vi "Save Values_UI.vi"(8 "error in (no error)":errorcluster, 10 "Controls and Indicators\nReferences":T1, 11 "Input ListBox Cluster":T7) -> (0 "error out":errorcluster, 3 "ListBox Cluster out":T7)   [LabVIEW 2019, in "ZenGage v3.0 UI.lvclass"]
doc: "This VI replaces entered Lower Limit, Upper Limit, Lower Control Limit, and Upper Control Limit in Measurement Listbox and Edit Measurement Listbox and then sends message to Save pressed_SM.vi."
uses:
  ZenGage v3.0 UI.lvclass
  Type Definitions/Edit tolerance settings/Rack Selection.ctl
  Type Definitions/Edit tolerance settings/Edit Tolerance Input.ctl
  <vilib>/Utility/miscctls.llb/LVPoint32TypeDef.ctl
  Type Definitions/Controls and Indicators/Select a part (combobox).ctl
  Type Definitions/Controls and Indicators/EDL control references.ctl
  Type Definitions/Controls and Indicators/Diagnostics control referencs.ctl
  Type Definitions/Controls and Indicators/Inspection control references.ctl
  Type Definitions/Controls and Indicators/General_Control references.ctl
  Type Definitions/Controls and Indicators/Controls and Indicators Cluster.ctl
  Type Definitions/General/Master sample references.ctl
panel:
  in  "Rack Number":i32
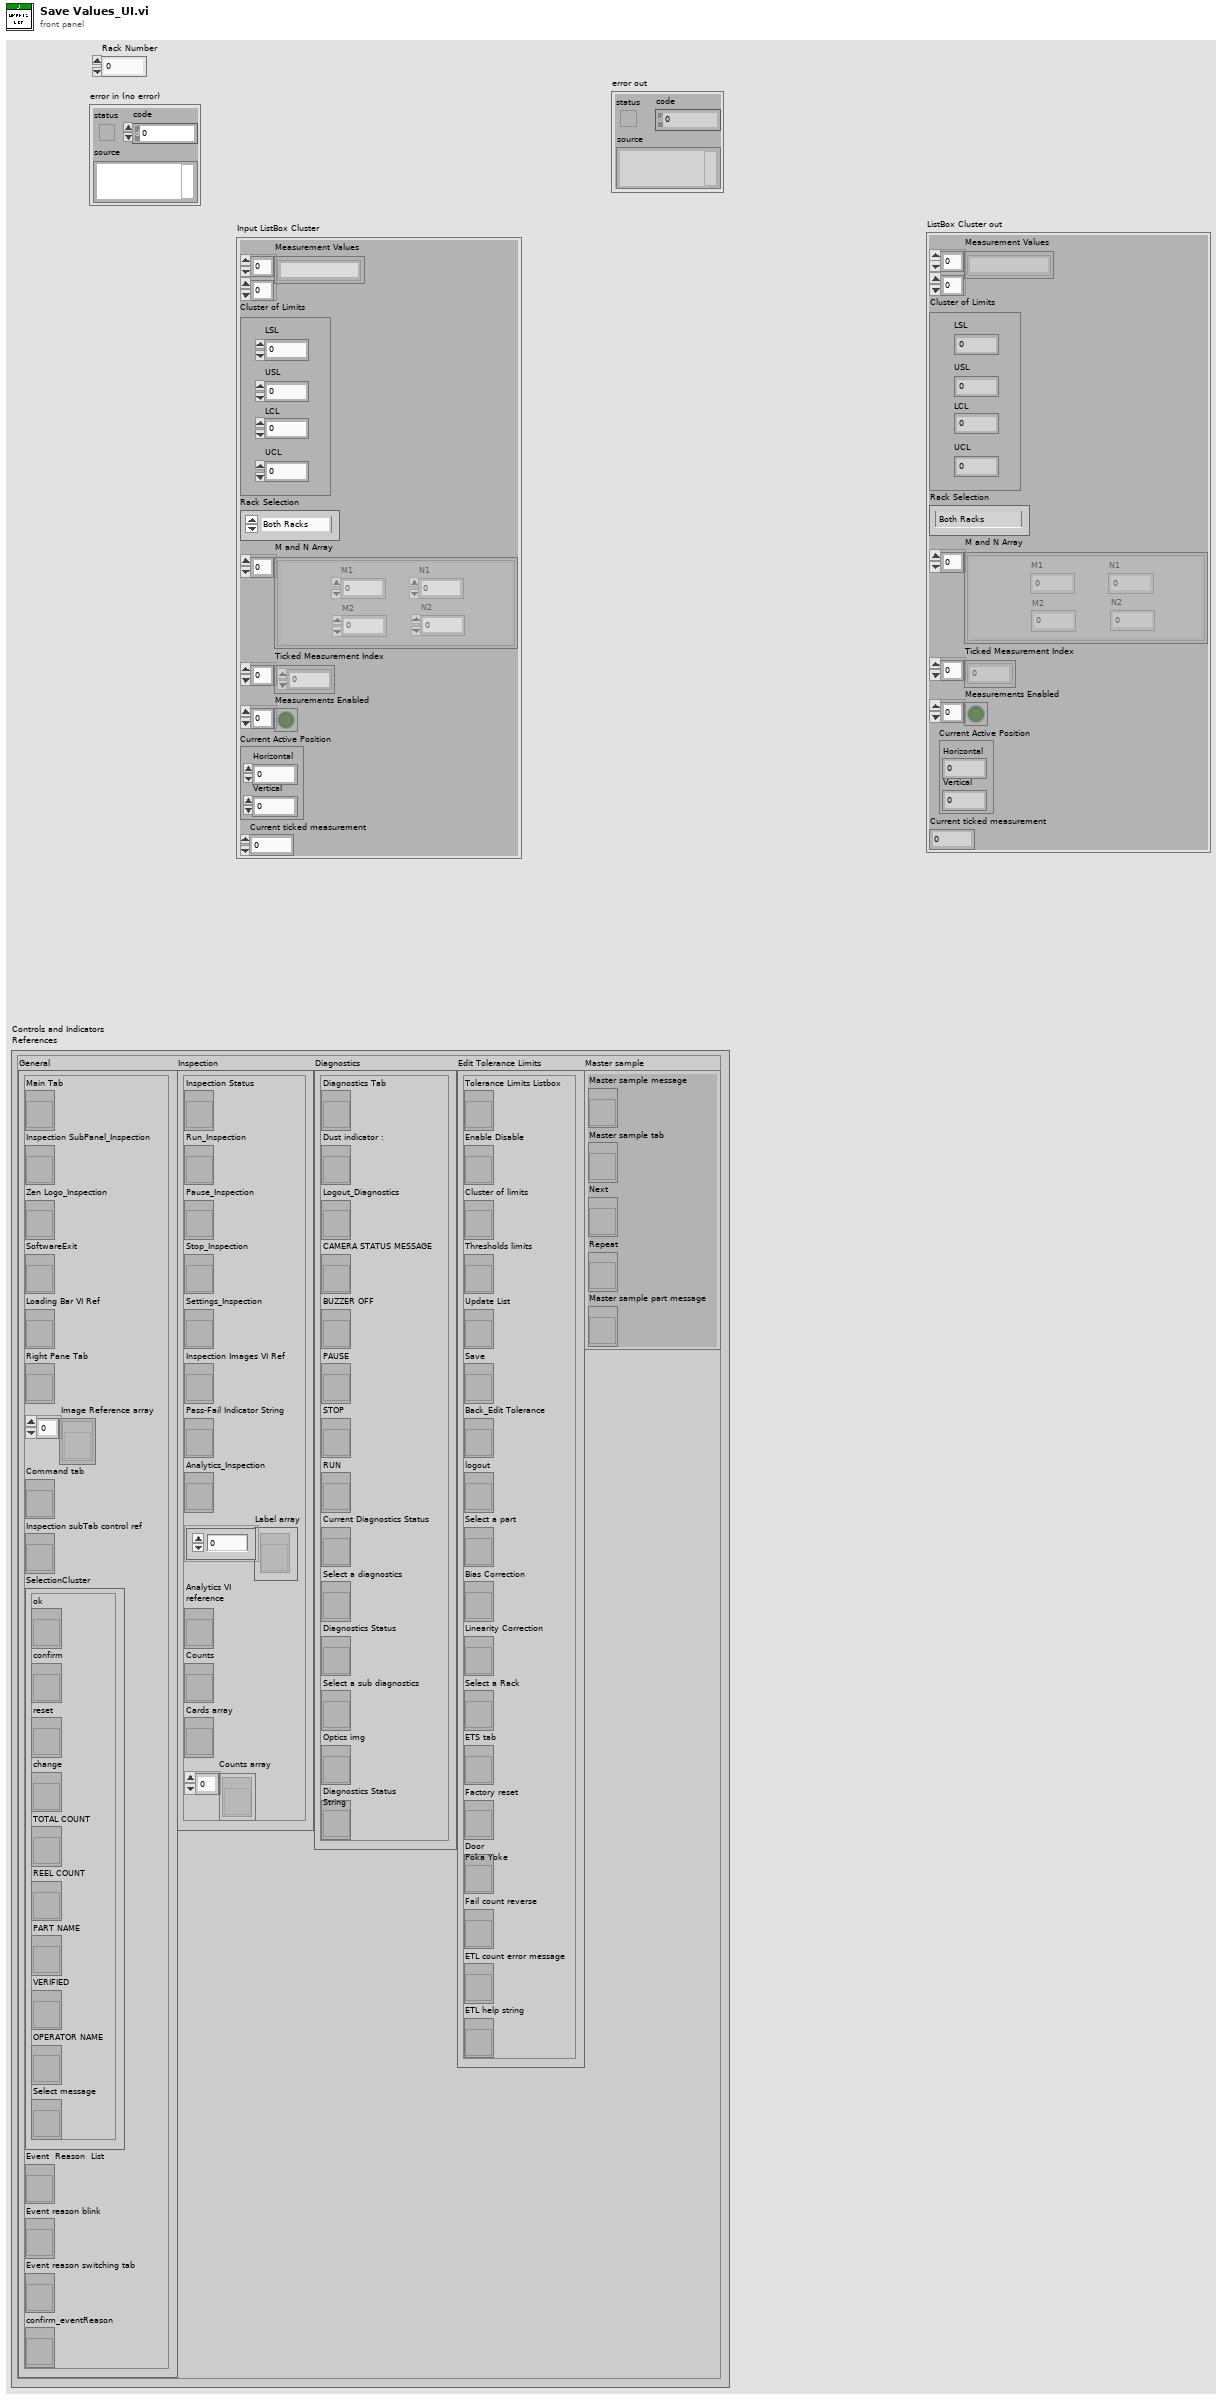
[diagram p1: front panel]
types:
  T1 = typedef "ZenGage v3.0 UI.lvclass/Controls and Indicators Cluster.ctl" = cluster{"General":T2, "Inspection":T3, "Diagnostics":T4, "Edit Tolerance Limits":T5, "Master sample":T6}
  T2 = typedef "ZenGage v3.0 UI.lvclass/General_Control references.ctl" = cluster{"Main Tab":refnum<vi>, "Inspection SubPanel_Inspection":refnum<vi>, "Zen Logo_Inspection":refnum<vi>, "SoftwareExit":refnum<vi>, "Loading Bar VI Ref":refnum<vi>, "Right Pane Tab":refnum<vi>, "Image Reference array":refnum<vi>[], "Command tab":refnum<vi>, "Inspection subTab control ref":refnum<vi>, "SelectionCluster":cluster{"ok":refnum<vi>, "confirm":refnum<vi>, "reset":refnum<vi>, "change":refnum<vi>, "TOTAL COUNT":refnum<vi>, "REEL COUNT":refnum<vi>, "PART NAME":refnum<vi>, "VERIFIED":refnum<vi>, "OPERATOR NAME":refnum<vi>, "Select message":refnum<vi>}, "Event  Reason  List":refnum<vi>, "Event reason blink":refnum<vi>, "Event reason switching tab":refnum<vi>, "confirm_eventReason":refnum<vi>}
  T3 = typedef "ZenGage v3.0 UI.lvclass/Inspection control references.ctl" = cluster{"Inspection Status":refnum<vi>, "Run_Inspection":refnum<vi>, "Pause_Inspection":refnum<vi>, "Stop_Inspection":refnum<vi>, "Settings_Inspection":refnum<vi>, "Inspection Images VI Ref":refnum<vi>, "Pass-Fail Indicator String":refnum<vi>, "Analytics_Inspection":refnum<vi>, "Label array":refnum<vi>[], "Analytics VI\nreference":refnum<vi>, "Counts":refnum<vi>, "Cards array":refnum<vi>, "Counts array":refnum<vi>[]}
  T4 = typedef "ZenGage v3.0 UI.lvclass/Diagnostics control referencs.ctl" = cluster{"Diagnostics Tab":refnum<vi>, "Dust indicator :":refnum<vi>, "Logout_Diagnostics":refnum<vi>, "CAMERA STATUS MESSAGE":refnum<vi>, "BUZZER OFF":refnum<vi>, "PAUSE":refnum<vi>, "STOP":refnum<vi>, "RUN":refnum<vi>, "Current Diagnostics Status":refnum<vi>, "Select a diagnostics":refnum<vi>, "Diagnostics Status":refnum<vi>, "Select a sub diagnostics":refnum<vi>, "Optics img":refnum<vi>, "Diagnostics Status\nString":refnum<vi>}
  T5 = typedef "ZenGage v3.0 UI.lvclass/EDL control references.ctl" = cluster{"Tolerance Limits Listbox":refnum<vi>, "Enable Disable":refnum<vi>, "Cluster of limits":refnum<vi>, "Thresholds limits":refnum<vi>, "Update List":refnum<vi>, "Save":refnum<vi>, "Back_Edit Tolerance":refnum<vi>, "logout":refnum<vi>, "Select a part":refnum<vi>, "Bias Correction":refnum<vi>, "Linearity Correction":refnum<vi>, "Select a Rack":refnum<vi>, "ETS tab":refnum<vi>, "Factory reset":refnum<vi>, "Door\nPoka Yoke":refnum<vi>, "Fail count reverse":refnum<vi>, "ETL count error message":refnum<vi>, "ETL help string":refnum<vi>}
  T6 = typedef "Master sample references.ctl" = cluster{"Master sample message":refnum<vi>, "Master sample tab":refnum<vi>, "Next":refnum<vi>, "Repeat":refnum<vi>, "Master sample part message":refnum<vi>}
  T7 = typedef "ZenGage v3.0 UI.lvclass/Edit Tolerance Input.ctl" = cluster{"Measurement Values":string[][], "Cluster of Limits":cluster{"LSL":dbl, "USL":dbl, "LCL":dbl, "UCL":dbl}, "Rack Selection":T8, "M and N Array":cluster{"M1":u64, "M2":u64, "N1":u64, "N2":u64}[], "Ticked Measurement Index":u32[], "Measurements Enabled":bool[], "Current Active Position":T9, "Current ticked measurement":dbl}
  T8 = typedef "ZenGage v3.0 UI.lvclass/Rack Selection.ctl" = enum16{"Both Racks", "Rack 2", "Rack 1"}
  T9 = typedef "LVPoint32TypeDef.ctl" = cluster{"Horizontal":i32, "Vertical":i32}
  T10 = enum8{"Enabled", "Disabled", "Disabled and Grayed Out"}
  T11 = cluster{"Lower Limit":dbl, "Upper Limit":dbl, "Lower Control Limit":dbl, "Upper Control Limit":dbl}
  T12 = cluster{"Control Limit Fail Allowable":u64, "Control Limit Fail Window":u64, "Spec Limit Fail Allowable":u64, "Spec Limit Fail Window":u64}
  T13 = cluster{"LSL":dbl, "USL":dbl, "LCL":dbl, "UCL":dbl}
  T14 = cluster{"M1":u64, "M2":u64, "N1":u64, "N2":u64}[]
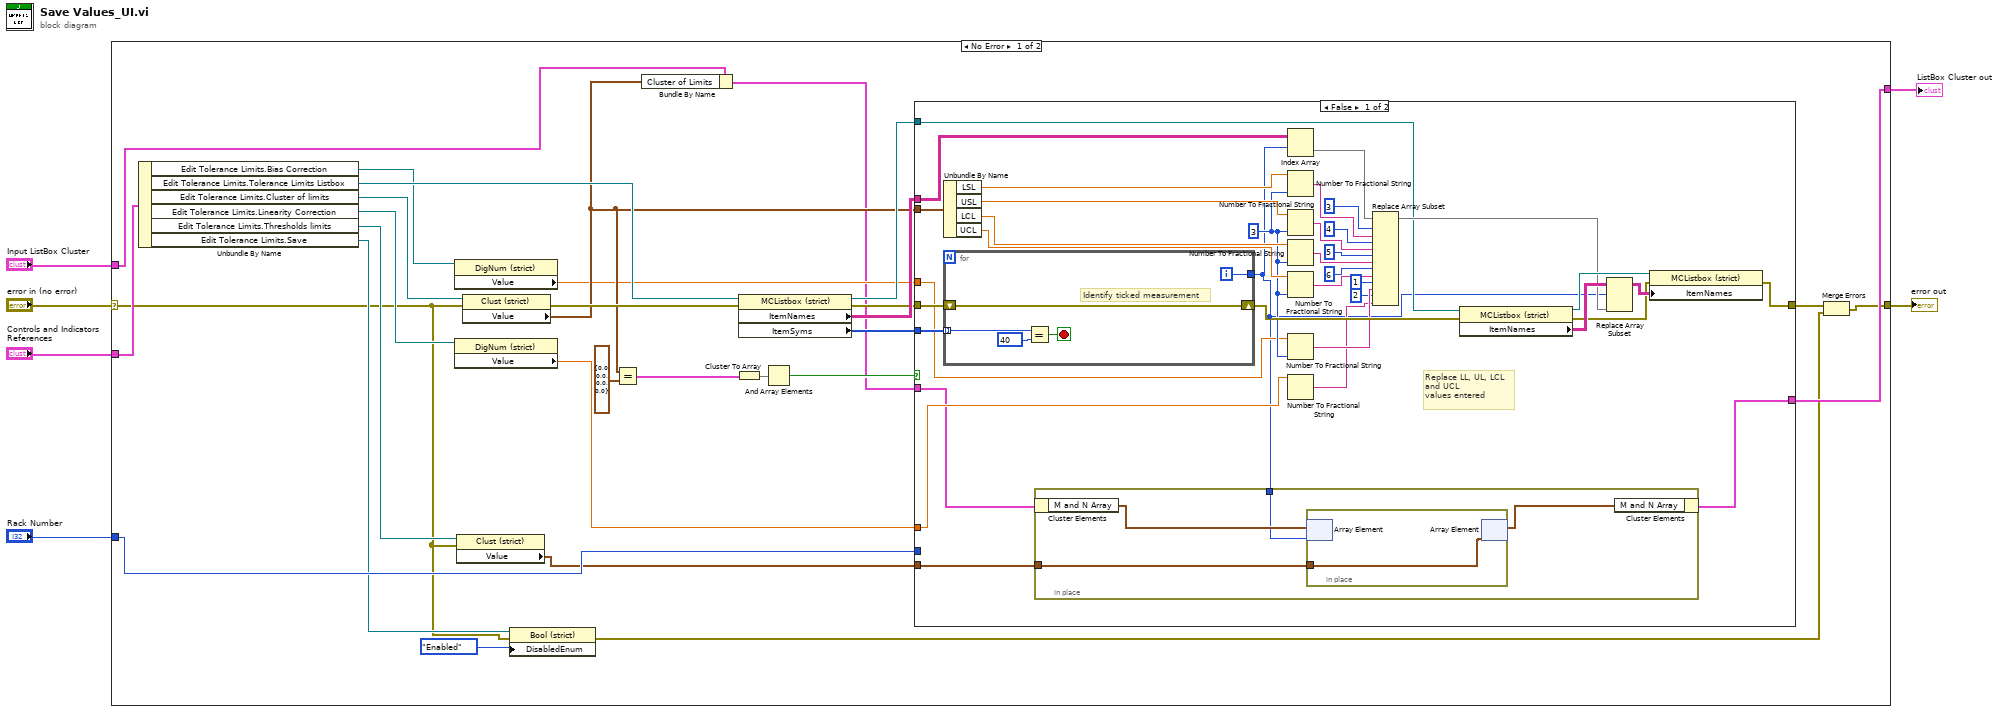
[diagram p0: block diagram]
diagram:
  n1 = case shown="No Error" "error in (no error)" {
    selector: "error in (no error)" -> [w10 w85]
    tunnel: [w7 w85] -> w5
    tunnel: "Input ListBox Cluster" -> [w13 w84]
    tunnel: [w14 w84] -> w3
    tunnel: "Rack Number" -> [w17 _]
    tunnel: "Controls and Indicators\nReferences" -> [w18 _]
    frame No Error {
      n2 = Unbundle By Name(w18) -> ("Edit Tolerance Limits.Bias Correction"=w23:refnum<vi>, "Edit Tolerance Limits.Tolerance Limits Listbox"=w25:refnum<vi>, "Edit Tolerance Limits.Cluster of limits"=w27:refnum<vi>, "Edit Tolerance Limits.Linearity Correction"=w21:refnum<vi>, "Edit Tolerance Limits.Thresholds limits"=w19:refnum<vi>, "Edit Tolerance Limits.Save"=w12:refnum<vi>)
      n3 = property class="DigNum (strict)"(reference=w23) -> ("Value"=w22:dbl)  [unwired: 1 in, 2 out]
      n4 = property class="DigNum (strict)"(reference=w21) -> ("Value"=w20:dbl)  [unwired: 1 in, 2 out]
      n5 = property class="Clust (strict)"(reference=w19, error in=w10) -> ("Value"=w16:T12)  [unwired: 2 out]
      n6 = property class="Clust (strict)"(reference=w27, error in=w10) -> (error out=w26:errorcluster, "Value"=w24:T13)  [unwired: 1 out]
      n7 = property class="Bool (strict)"(reference=w12, error in=w10, "DisabledEnum"=T10."Enabled" ("Disabled")) -> (error out=w8:errorcluster)  [unwired: 1 out]
      n8 = Equal?(x=w24, y=T11 {"Lower Limit"=0.0, "Upper Limit"=0.0, "Lower Control Limit"=0.0, "Upper Control Limit"=0.0} ("Value")) -> (x = y?=w33:cluster{bool, bool, bool, bool})
      n9 = Bundle By Name(cluster=w13, "Cluster of Limits"=w24) -> (w15:T7)
      n10 = Cluster To Array(cluster=w33) -> (array=w34:bool[])
      n11 = property class="MCListbox (strict)"(reference=w25, error in=w26) -> (reference out=w28:refnum<vi>, error out=w30:errorcluster, "ItemNames"=w31:string[][], "ItemSyms"=w29:i32[])
      n12 = And Array Elements(Boolean array=w34) -> (logical AND=w35:bool)
      n13 = case shown="False" w35 {
        tunnel: w29 -> [w71 _]
        tunnel: w28 -> [w40 _]
        tunnel: w30 -> [w51 w83]
        tunnel: [w49 w83] -> w9
        tunnel: w31 -> [w56 _]
        tunnel: w24 -> [w52 _]
        tunnel: w22 -> [w46 _]
        tunnel: w20 -> [w42 _]
        tunnel: w17 -> [_ _]
        tunnel: w16 -> [w39 _]
        tunnel: w15 -> [w37 w82]
        tunnel: [w36 w82] -> w14
        frame False {
          w47 = i16 3 ("precision (6)")
          # "Replace LL, UL, LCL \nand UCL\nvalues entered"
          n14 = Unbundle By Name(w52) -> ("LSL"=w69:dbl, "USL"=w68:dbl, "LCL"=w67:dbl, "UCL"=w66:dbl)
          n15 = for {
            tunnel: w71 -> [w80] mode=indexing
            tunnel: [w78] -> w38
            shift-right: [w77] -> w50
            shift-left: w51 -> [w77]
            i -> [w78]
            stop <- w79 stop-if-true
            # "Identify ticked measurement"
            n16 = Equal?(x=w80, y=40) -> (x = y?=w79:bool)
          }
          n17 = in-place {
            in-place-border: w39 -> [w75]
            in-place-border: w38 -> [w72]
            n18 = in-place-cluster #1(w37) -> ("M and N Array"=w74:T14)
            n19 = in-place {
              in-place-border: w75 -> [w76]
              n20 = in-place-array #2(w74, w72) -> ()  [unwired: 1 out]
              n21 = in-place-array #2(w76) -> (w73:T14)  [unwired: 1 out]
            }
            n22 = in-place-cluster #1("M and N Array"=w73) -> (w36:T7)
          }
          n23 = Index Array(array=w56, index (row)=w38) -> (element=w70:string[])  [unwired: 1 in]
          n24 = Number To Fractional String(number=w69, precision (6)=w47) -> (F-format string=w65:string)  [unwired: 2 in]
          n25 = Number To Fractional String(number=w68, precision (6)=w47) -> (F-format string=w64:string)  [unwired: 2 in]
          n26 = Number To Fractional String(number=w67, precision (6)=w47) -> (F-format string=w63:string)  [unwired: 2 in]
          n27 = Number To Fractional String(number=w66, precision (6)=w47) -> (F-format string=w62:string)  [unwired: 2 in]
          n28 = Number To Fractional String(number=w46, precision (6)=w47) -> (F-format string=w44:string)  [unwired: 2 in]
          n29 = Number To Fractional String(number=w42) -> (F-format string=w41:string)  [unwired: 3 in]
          n30 = Replace Array Subset(array=w70, new element #1=w65, index #1=3 ("index"), new element #2=w64, index #2=4 ("index"), new element #3=w63, index #3=5 ("index"), new element #4=w62, index #4=6 ("index"), new element #5=w44, index #5=1 ("index"), new element #6=w41, index #6=2 ("index")) -> (w53:string[])
          n31 = property class="MCListbox (strict)"(reference=w40, error in=w50) -> (reference out=w57:refnum<vi>, error out=w48:errorcluster, "ItemNames"=w55:string[][])
          n32 = Replace Array Subset(array=w55, new element=w53, index (row)=w38) -> (w54:string[][])  [unwired: 1 in]
          n33 = property class="MCListbox (strict)"(reference=w57, error in=w48, "ItemNames"=w54) -> (error out=w49:errorcluster)  [unwired: 1 out]
        }
        frame True {
        }
      }
      n34 = Merge Errors(w9, w8) -> (w7:errorcluster)
    }
    frame Error {
    }
  }
  "error out" <- w5
  "ListBox Cluster out" <- w3
